vi "UT_LokiJsonFormatter_Main.vi"(8 "error in":errorcluster) -> (0 "error out":errorcluster)   [LabVIEW 2017, in "UT_LokiJsonFormatter.lvlib"]
uses:
  UT_LokiJsonFormatter.lvlib
  <vilib>/addons/_JKI Toolkits/Caraya/classes/Test/Test.lvclass
panel:
  # "Connector Pane"
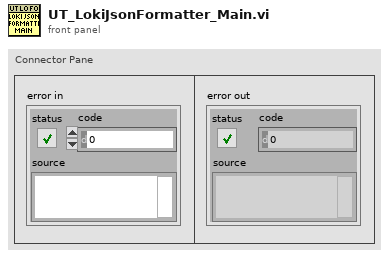
[diagram p1: front panel]
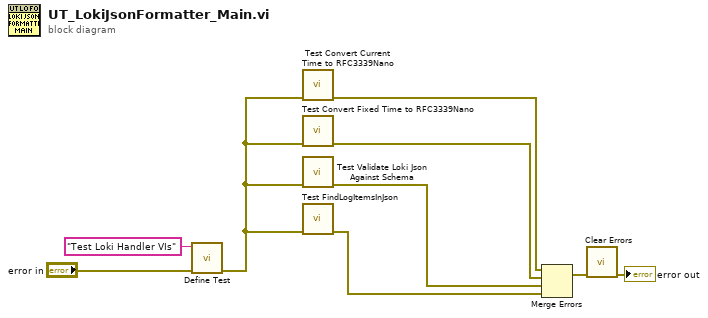
[diagram p0: block diagram]
diagram:
  n1 = call <vilib>:"Define Test.vi"("error in (no error)"="error in", "Label (VI Title)"="Test Loki Handler VIs") -> ("error out"=w1:errorcluster)  [unwired: 8 in, 1 out]
  n2 = call "Test Convert Current Time to RFC3339Nano.vi"("error in (no error)"=w1) -> ("error out"=w7:errorcluster)  [unwired: 10 in]
  n3 = call "Test Convert Fixed Time to RFC3339Nano.vi"("error in (no error)"=w1) -> ("error out"=w6:errorcluster)  [unwired: 10 in]
  n4 = call "Test Validate Loki Json Against Schema.vi"("error in (no error)"=w1) -> ("error out"=w3:errorcluster)  [unwired: 10 in]
  n5 = call "Test FindLogItemsInJson.vi"("error in (no error)"=w1) -> ("error out"=w2:errorcluster)  [unwired: 10 in]
  n6 = Merge Errors(w7, w6, w3, w2) -> (w4:errorcluster)
  n7 = call <vilib>:"Clear Errors.vi"("error in (no error)"=w4) -> ("error out"=→"error out":errorcluster)  [unwired: 5 in, 1 out]
